vi "Wrist (SubVI).vi"(0 "Call Context":refnum<vi>, 1 "Wrist Invert Motor Limit":bool, 2 "Wrist Setpoints":dbl[](array[numeric])=[-7000.0, -7000.0, 80000.0, 70000.0, 136000.0, 45000.0, 29000.0, 65000.0, -65000.0], 3 "Wrist Invert Encoder Limit":bool, 4 "Wrist PID Gains":T2={"proportional gain (Kc)"=2e-05, "integral time (Ti, min)"=0.0, "derivative time (Td, min)"=0.0}, 6 "Wrist Output Range":cluster{"output high":dbl, "output low":dbl}={"output high"=0.5, "output low"=-0.5}, 7 "Setpoint \nOverride":bool, 8 "Wrist Setpoint ID":T1(ring), 9 "Safety Override":bool, 10 "Intake Encoder Limit":dbl=110000.0 format="%#_13g", 11 "Override Power":dbl, 12 "Intake Home Encoder Limit":dbl=-45000.0 format="%#_13g", 13 "Wrist Auto":bool=TRUE) -> (14 "Wrist Hold Position":i32, 15 "Switch Pressed":bool)   [LabVIEW 2018]
uses:
  <vilib>/Rock Robotics/WPI/ThirdParty/Phoenix-LabVIEW/Motor Controller/Controls/CTRE_Phoenix_MotorControl_ControlMode.ctl
  <vilib>/Rock Robotics/WPI/DriverStation/WPI_DriverStationDerivedRobotMode.ctl
  <vilib>/Rock Robotics/WPI/ThirdParty/Phoenix-LabVIEW/Motor Controller/Get/CTRE_Phoenix_MotorController_GetSelectedSensorData.vi
  Toolbox/Simple Limit Switch/Limits(DoubleEncoder).vi
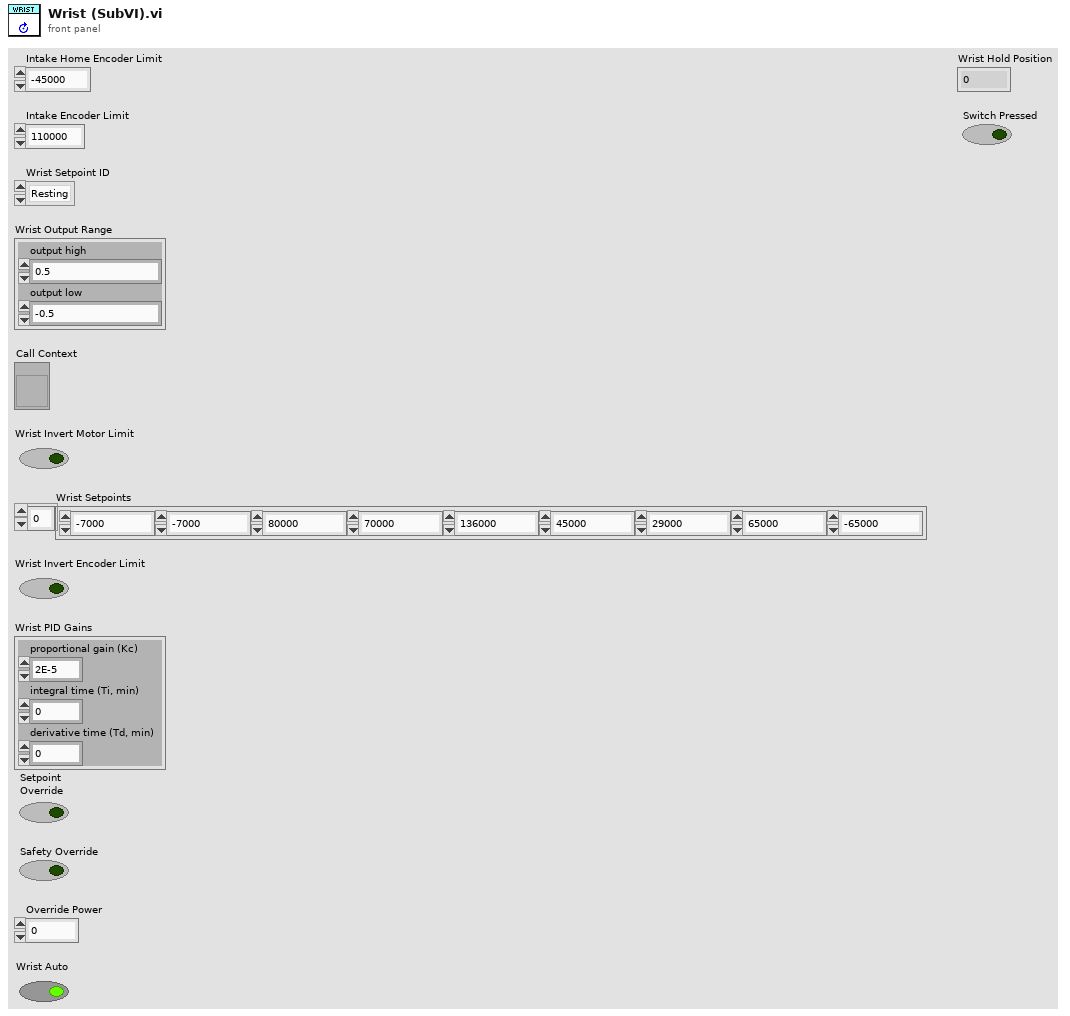
[diagram p1: front panel]
types:
  T1 = enum16{"Resting", "Hatch Ground Intake", "Hatch Place Low/Mid/CargoShip", "Hatch Place High", "Cargo Ground Intake", "Cargo Place Low/Mid", "Cargo Place High", "CargoShip Place Front", "CargoShip Place Back"}
  T2 = cluster{"proportional gain (Kc)":dbl, "integral time (Ti, min)":dbl, "derivative time (Td, min)":dbl}
  T3 = typedef "WPI_DriverStationDerivedRobotMode.ctl" = enum16{"Init", "Execute", "Stop"}
  T4 = typedef "CTRE_Phoenix_MotorControl_ControlMode.ctl" = u16
  T5 = typedef "WPI_SwitchDevRef.ctl" = cluster{"DevStatus":errorcluster, "DIO Channel":T6, "CntIndex":T7, "Normally Closed":bool}
  T6 = typedef "FPGA_DIOChannel.ctl" = enum8{"DIO 0", "DIO 1", "DIO 2", "DIO 3", "DIO 4", "DIO 5", "DIO 6", "DIO 7", "DIO 8", "DIO 9", "DIO MXP 0", "DIO MXP 1", "DIO MXP 2", "DIO MXP 3", "DIO MXP 4", "DIO MXP 5", "DIO MXP 6", "DIO MXP 7", "DIO MXP 8", "DIO MXP 9", "DIO MXP 10", "DIO MXP 11", "DIO MXP 12", "DIO MXP 13", "DIO MXP 14", "DIO MXP 15", "SPI Port CS1", "SPI Port CS2", "SPI Port CS3", "SPI Port MISO", "SPI Port MOSI", "Invalid"}
  T7 = typedef "FPGA_CounterCtrSystemIndex.ctl" = enum8{"Ctr 0", "Ctr 1", "Ctr 2", "Ctr 3", "Ctr 4", "Ctr 5", "Ctr 6", "Ctr 7", "Invalid"}
  T8 = typedef "WPI_MotorControlDeviceRef.ctl" = cluster{"DeviceStatus":errorcluster, "Type":T9, "PWM":cluster{"PWM Channel":T10, "DeadBand":T11}, "CAN":cluster{"Device Number":u8, "SetOutput VI Ref":variant, "GetOutput VI Ref":variant, "Enable VI Ref":variant, "Disable VI Ref":variant, "Data":variant}, "Invert":bool, "DIO PWM":cluster{"PWM \"Enable\" Channel":T10, "DIOChannel":T6, "PWM Rate":dbl}}
  T9 = typedef "WPI_MotorControlType.ctl" = enum16{"PWM", "CAN", "DIO PWM"}
  T10 = typedef "FPGA_DIOPWMChannel.ctl" = enum8{"PWM 0", "PWM 1", "PWM 2", "PWM 3", "PWM 4", "PWM 5", "PWM 6", "PWM 7", "PWM 8", "PWM 9", "PWM MXP 0", "PWM MXP 1", "PWM MXP 2", "PWM MXP 3", "PWM MXP 4", "PWM MXP 5", "PWM MXP 6", "PWM MXP 7", "PWM MXP 8", "PWM MXP 9", "Invalid"}
  T11 = typedef "WPI_PWMDeadband.ctl" = cluster{"Name":string, "maxPositivePwm":i32, "minPositivePwm":i32, "centerPwm":i32, "maxNegativePwm":i32, "minNegativePwm":i32, "angularRange":u16}
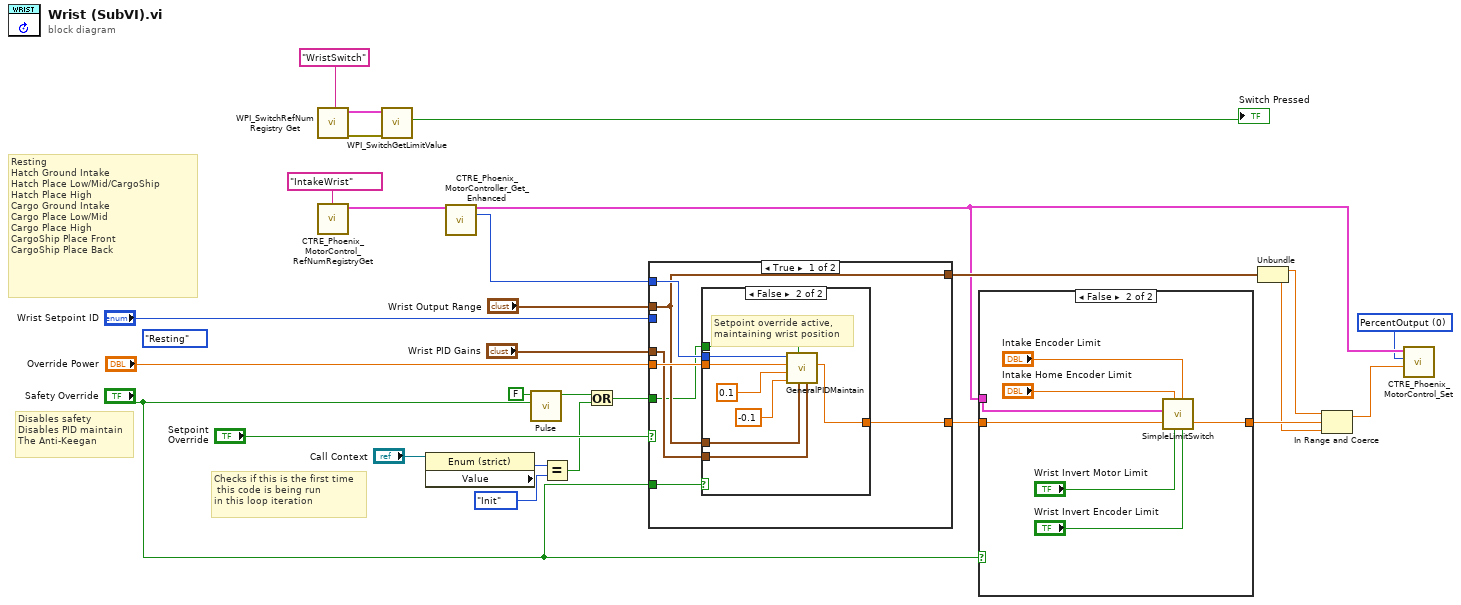
[diagram p0: block diagram]
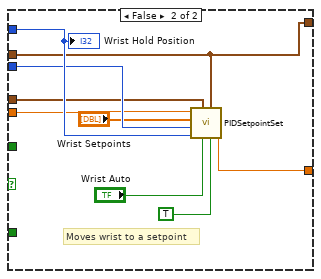
[diagram p3: hidden frame]
diagram:
  (unwired) T1."Resting" ("Wrist Setpoint ID")
  w9 = T4 0 items=["PercentOutput"=0, "Position"=1, "Velocity"=2, "Current"=3, "Follower"=5, "MotionProfile"=6, "MotionMagic"=7, "MotionProfileArc"=10, "Disabled"=15] ("Control Mode")
  # "Checks if this is the first time\n this code is being run \nin this loop iteration"
  # "Disables safety\nDisables PID maintain\nThe Anti-Keegan"
  # "Resting\nHatch Ground Intake\nHatch Place Low/Mid/CargoShip\nHatch Place High\nCargo Ground Intake\nCargo Place Low/Mid\nCargo Place High\nCargoShip Place Front\nCargoShip Place Back"
  n1 = call <vilib>:"WPI_SwitchRefNum Registry Get.vi"("refnum name"="WristSwitch") -> ("error out"=w4:errorcluster, "SwitchDevRef"=w5:T5)  [unwired: 9 in]
  n2 = call <vilib>:"CTRE_Phoenix_MotorControl_RefNumRegistryGet.vi"("refnum name"="IntakeWrist") -> ("PhoenixMotorControlDevRef"=w8:T8)  [unwired: 9 in, 1 out]
  n3 = call <vilib>:"WPI_SwitchGetLimitValue.vi"("error in (no error)"=w4, "SwitchDevRef"=w5) -> ("Switch Pressed"=→"Switch Pressed":bool)  [unwired: 7 in, 2 out]
  n4 = property class="Enum (strict)"(reference="Call Context") -> ("Value"=w23:T3)  [unwired: 1 in, 2 out]
  n5 = call-poly <vilib>:"CTRE_Phoenix_MotorController_Get_Enhanced.vi"("PhoenixMotorControlDevRef"=w8) -> ("PhoenixMotorControlDevRef"=w10:T8, "Position (Raw Sensor Units)"=w7:i32)  [unwired: 11 in, 2 out]
  n6 = call "Pulse.vi"("Input"="Safety Override", "Rising Edge?"=FALSE) -> ("Output"=w25:bool)  [unwired: 9 in]
  n7 = Equal?(x=w23, y=WPI_DriverStationDerivedRobotMode."Init") -> (x = y?=w27:bool)
  n8 = Or(x=w25, y=w27) -> (x .or. y?=w26:bool)
  n9 = case shown="True" "Setpoint \nOverride" {
    tunnel: w7 -> [w33 w53]
    tunnel: "Wrist Setpoint ID" -> [_ w52]
    tunnel: [w34 w50] -> w13
    tunnel: "Override Power" -> [w35 w48]
    tunnel: [w31 w45] -> w16
    tunnel: "Wrist PID Gains" -> [w32 w46]
    tunnel: "Wrist Output Range" -> [w31 w45]
    tunnel: "Safety Override" -> [w30 _]
    tunnel: w26 -> [w29 _]
    frame True {
      n10 = case shown="False" w30 {
        tunnel: w35 -> [w36 w44]
        tunnel: [w36 w43] -> w34
        tunnel: w33 -> [_ w42]
        tunnel: w32 -> [_ w39]
        tunnel: w31 -> [_ w38]
        tunnel: w29 -> [_ w37]
        frame True {
          # "Both overrides active, only override power"
        }
        frame False {
          # "Setpoint override active,\nmaintaining wrist position"
          n11 = call "GeneralPIDMaintain.vi"("PID gains"=w39, "Output Range"=w38, "Initialize"=w37, "Lower Power Limit"=-0.1, "Upper Power Limit"=0.1, "Power"=w44, "Encoder Position"=w42) -> ("Power Out"=w43:dbl)  [unwired: 4 in]
        }
      }
    }
    frame False {
      # "Moves wrist to a setpoint"
      n12 = call "PIDSetpointSet.vi"("Update"=TRUE, "Output Range"=w45, "Auto"="Wrist Auto", "PID Gains"=w46, "Encoder Position"=w53, "Level"=w52, "Setpoints"="Wrist Setpoints", "Manual Power"=w48) -> ("Power Out"=w50:dbl)  [unwired: 3 in]
      "Wrist Hold Position" <- w53
    }
  }
  n13 = case shown="False" "Safety Override" {
    tunnel: [w54 w61] -> w19
    tunnel: w10 -> [_ w60]
    tunnel: w13 -> [w54 w55]
    frame True {
    }
    frame False {
      n14 = call-poly "SimpleLimitSwitch.vi"("Into Home Limit is Pos (Encoder)"="Wrist Invert Encoder Limit", "Encoder Limit"="Intake Encoder Limit", "Into Home Limit Is Pos (Motor)"="Wrist Invert Motor Limit", "Home Encoder Limit"="Intake Home Encoder Limit", "Power In"=w55, "Motor Ref"=w60) -> ("Power Out"=w61:dbl)  [unwired: 5 in]
    }
  }
  n15 = Unbundle(w16) -> ("output high"=w17:dbl, "output low"=w18:dbl)
  n16 = In Range and Coerce(upper limit=w17, x=w19, lower limit=w18) -> (coerced(x)=w15:dbl)  [unwired: 1 out]
  n17 = call <vilib>:"CTRE_Phoenix_MotorControl_Set.vi"("Output"=w15, "Control Mode"=w9, "PhoenixMotorControlDevRef"=w10) -> ()  [unwired: 7 in, 2 out]
